vi "Endianness.vi"() -> ()   [LabVIEW 2016]
panel:
  out "*(type *) &x 3":u64
  out "U8 7":bool[](array[boolean])
  out "U8 6":bool[](array[boolean])
  out "U8 5":bool[](array[boolean])
  out "U8 4":bool[](array[boolean])
  out "U8 3":bool[](array[boolean])
  out "U8 2":bool[](array[boolean])
  out "U8 1":bool[](array[boolean])
  out "U8 0":bool[](array[boolean])
  out "U64":bool[](array[boolean])
  out "*(type *) &x 2":u8[](array[numeric])
  out "*(type *) &x":u64[](array[numeric])
  in  "DBL":dbl
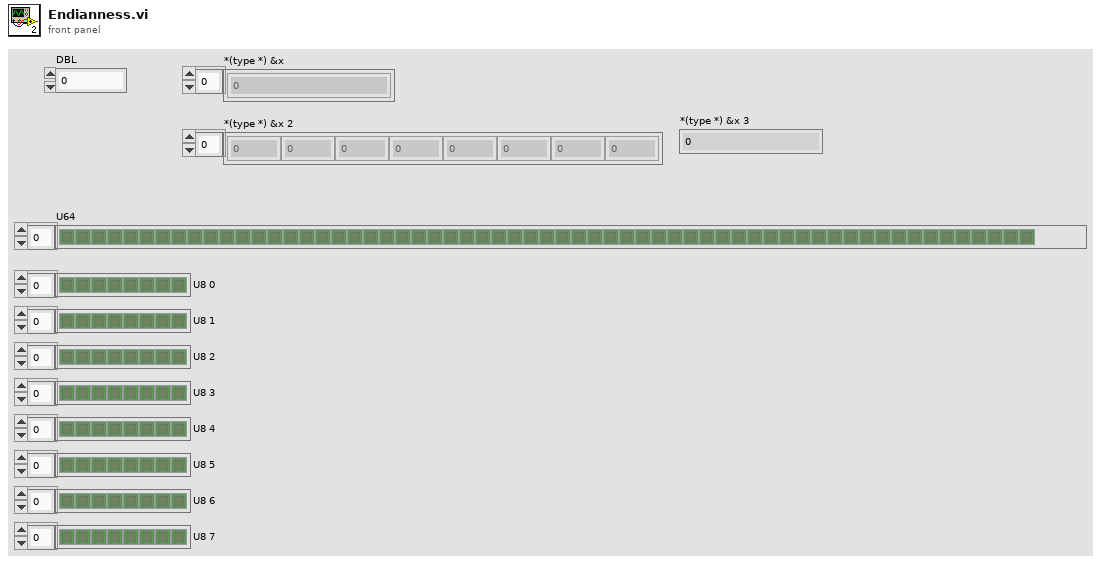
[diagram p1: front panel]
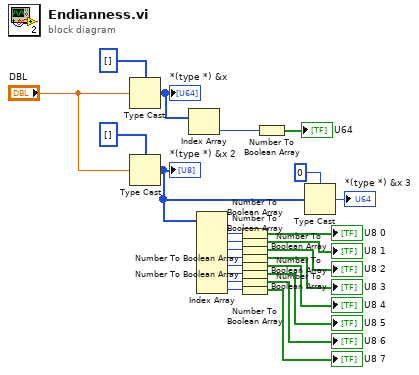
[diagram p0: block diagram]
diagram:
  n1 = Type Cast(type=u64[] [], x="DBL") -> (*(type *) &x=w23:u64[])
  "*(type *) &x" <- w23
  n2 = Type Cast(type=u8[] [], x="DBL") -> (*(type *) &x=w4:u8[])
  "*(type *) &x 2" <- w4
  n3 = Index Array(array=w23) -> (element=w22:u64)  [unwired: 1 in]
  n4 = Index Array(array=w4) -> (element #1=w20:u8, element #2=w19:u8, element #3=w18:u8, element #4=w17:u8, element #5=w16:u8, element #6=w15:u8, element #7=w14:u8, element #8=w13:u8)  [unwired: 8 in]
  n5 = Number To Boolean Array(number=w20) -> (Boolean array=→"U8 0":bool[])
  n6 = Number To Boolean Array(number=w19) -> (Boolean array=→"U8 1":bool[])
  n7 = Number To Boolean Array(number=w18) -> (Boolean array=→"U8 2":bool[])
  n8 = Number To Boolean Array(number=w17) -> (Boolean array=→"U8 3":bool[])
  n9 = Number To Boolean Array(number=w16) -> (Boolean array=→"U8 4":bool[])
  n10 = Number To Boolean Array(number=w15) -> (Boolean array=→"U8 5":bool[])
  n11 = Number To Boolean Array(number=w14) -> (Boolean array=→"U8 6":bool[])
  n12 = Number To Boolean Array(number=w13) -> (Boolean array=→"U8 7":bool[])
  n13 = Number To Boolean Array(number=w22) -> (Boolean array=→"U64":bool[])
  n14 = Type Cast(type=u64 0, x=w4) -> (*(type *) &x=→"*(type *) &x 3":u64)
